vi "sub_joystick-data-conv.vi"(11 "joystick info-in":T1) -> (2 "cmd":u32, 3 "opval":cluster{dbl, dbl} {"?" format="%-1.1f"; "?" format="%-1.1f"})   [LabVIEW 2019]
uses:
  Ctrl/cmd_common.ctl
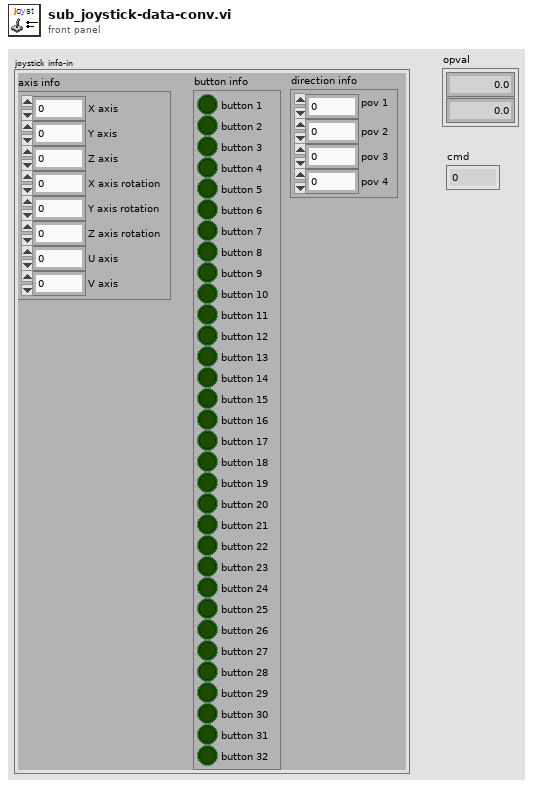
[diagram p1: front panel]
types:
  T1 = cluster{"axis info":cluster{"X axis":i32, "Y axis":i32, "Z axis":i32, "X axis rotation":i32, "Y axis rotation":i32, "Z axis rotation":i32, "U axis":i32, "V axis":i32}, "button info":cluster{"button 1":bool, "button 2":bool, "button 3":bool, "button 4":bool, "button 5":bool, "button 6":bool, "button 7":bool, "button 8":bool, "button 9":bool, "button 10":bool, "button 11":bool, "button 12":bool, "button 13":bool, "button 14":bool, "button 15":bool, "button 16":bool, "button 17":bool, "button 18":bool, "button 19":bool, "button 20":bool, "button 21":bool, "button 22":bool, "button 23":bool, "button 24":bool, "button 25":bool, "button 26":bool, "button 27":bool, "button 28":bool, "button 29":bool, "button 30":bool, "button 31":bool, "button 32":bool}, "direction info":cluster{"pov 1":i32, "pov 2":i32, "pov 3":i32, "pov 4":i32}}
  T2 = enum16{"none", "ERP42", "ERP42mini", "Scout", "Ycar"}
  T3 = typedef "cmd_common.ctl" = enum16{"read", "write"}
  T4 = typedef "joystick cfg.ctl" = cluster{"Type":enum16{"Logitech F710", "Xbox"}, "steer limit":cluster{"min":dbl, "max":dbl, "scale":dbl, "offset":dbl}, "speed limit":cluster{"min":dbl, "max":dbl, "pwm max":dbl}, "ID":i32, "joystick max":dbl}
  T5 = cluster{"button 1":bool, "button 2":bool, "button 3":bool, "button 4":bool, "button 5":bool, "button 6":bool, "button 7":bool, "button 8":bool, "button 9":bool, "button 10":bool, "button 11":bool, "button 12":bool, "button 13":bool, "button 14":bool, "button 15":bool, "button 16":bool, "button 17":bool, "button 18":bool, "button 19":bool, "button 20":bool, "button 21":bool, "button 22":bool, "button 23":bool, "button 24":bool, "button 25":bool, "button 26":bool, "button 27":bool, "button 28":bool, "button 29":bool, "button 30":bool, "button 31":bool, "button 32":bool}
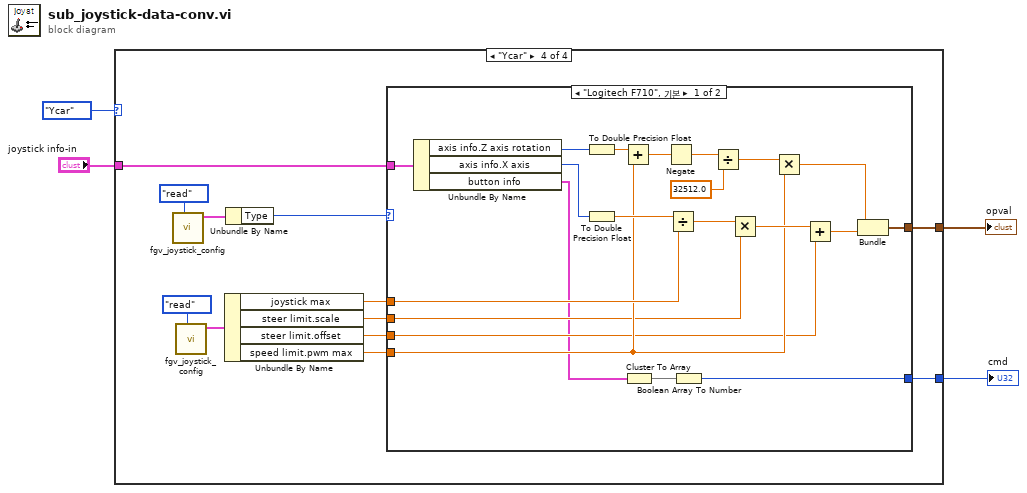
[diagram p0: block diagram]
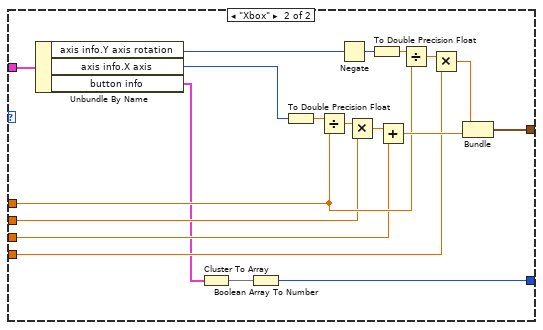
[diagram p5: hidden frame]
diagram:
  n1 = case shown="\"Ycar\"" T2."Ycar" ("AGV") {
    tunnel: [_ _ _ w16] -> w4
    tunnel: "joystick info-in" -> [_ _ _ w15]
    tunnel: [_ _ _ w5] -> w1
    frame "ERP42", Default {
    }
    frame "ERP42mini" {
    }
    frame "Scout" {
    }
    frame "Ycar" {
      n2 = call "fgv_joystick_config.vi"("cmd"=cmd_common."read") -> ("Joystick cfg out"=w13:T4)  [unwired: 9 in, 1 out]
      n3 = call "fgv_joystick_config.vi"("cmd"=cmd_common."read") -> ("Joystick cfg out"=w11:T4)  [unwired: 9 in, 1 out]
      n4 = Unbundle By Name(w11) -> ("joystick max"=w9:dbl, "steer limit.scale"=w8:dbl, "steer limit.offset"=w7:dbl, "speed limit.pwm max"=w6:dbl)
      n5 = Unbundle By Name(w13) -> ("Type"=w12:enum16{"Logitech F710", "Xbox"})
      n6 = case shown="\"Logitech F710\", 기본" w12 {
        tunnel: [w37 w47] -> w16
        tunnel: w15 -> [w27 w49]
        tunnel: w9 -> [w23 w44]
        tunnel: w8 -> [w21 w43]
        tunnel: w7 -> [w20 w42]
        tunnel: w6 -> [w22 w41]
        tunnel: [w17 w38] -> w5
        frame "Logitech F710", Default {
          n7 = Unbundle By Name(w27) -> ("axis info.Z axis rotation"=w26:i32, "axis info.X axis"=w32:i32, "button info"=w18:T5)
          n8 = To Double Precision Float(number=w26) -> (double precision float=w29:dbl)
          n9 = To Double Precision Float(number=w32) -> (double precision float=w28:dbl)
          n10 = Add(x=w29, y=w22) -> (x+y=w36:dbl)
          n11 = Cluster To Array(cluster=w18) -> (array=w19:bool[])
          n12 = Negate(x=w36) -> (-x=w34:dbl)
          n13 = Divide(x=w28, y=w23) -> (x/y=w31:dbl)
          n14 = Boolean Array To Number(Boolean array=w19) -> (number=w17:u32)
          n15 = Divide(x=w34, y=32512.0) -> (x/y=w33:dbl)
          n16 = Multiply(x=w31, y=w21) -> (x*y=w30:dbl)
          n17 = Multiply(x=w33, y=w22) -> (x*y=w25:dbl)
          n18 = Add(x=w30, y=w20) -> (x+y=w24:dbl)
          n19 = Bundle(w25, w24) -> (w37:cluster{dbl, dbl})  [unwired: 1 in]
        }
        frame "Xbox" {
          n20 = Unbundle By Name(w49) -> ("axis info.Y axis rotation"=w50:i32, "axis info.X axis"=w56:i32, "button info"=w40:T5)
          n21 = Cluster To Array(cluster=w40) -> (array=w39:bool[])
          n22 = Boolean Array To Number(Boolean array=w39) -> (number=w38:u32)
          n23 = To Double Precision Float(number=w56) -> (double precision float=w53:dbl)
          n24 = Divide(x=w53, y=w44) -> (x/y=w55:dbl)
          n25 = Negate(x=w50) -> (-x=w48:i32)
          n26 = Multiply(x=w55, y=w43) -> (x*y=w54:dbl)
          n27 = To Double Precision Float(number=w48) -> (double precision float=w52:dbl)
          n28 = Add(x=w54, y=w42) -> (x+y=w45:dbl)
          n29 = Divide(x=w52, y=w44) -> (x/y=w51:dbl)
          n30 = Multiply(x=w51, y=w41) -> (x*y=w46:dbl)
          n31 = Bundle(w46, w45) -> (w47:cluster{dbl, dbl})  [unwired: 1 in]
        }
      }
    }
  }
  "opval" <- w4
  "cmd" <- w1
